vi "Timer.vi"(11 "Error_In":errorcluster, 13 "Timer_Select":T1=enum."Time_Out?") -> (4 "Time_Out?":bool, 15 "Error_Out":errorcluster)   [LabVIEW 2021]
doc: "Used for time out opertion."
uses:
  Controls/Timer_Select.ctl
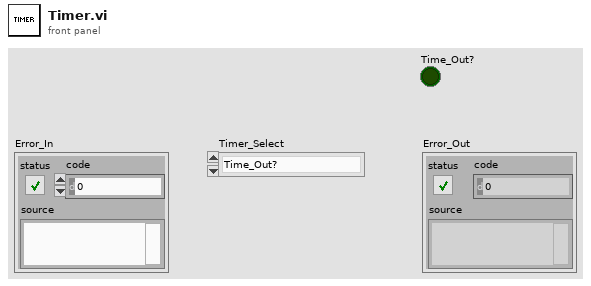
[diagram p1: front panel]
types:
  T1 = typedef "Timer_Select.ctl" = enum16{"Start_Timer", "Time_Out?", "Stop_Timer"}
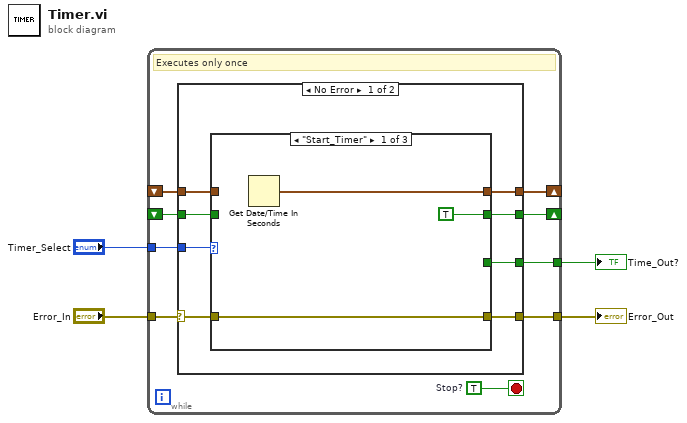
[diagram p0: block diagram]
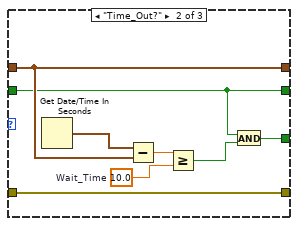
[diagram p2: hidden frame]
diagram:
  n1 = while {
    tunnel: "Timer_Select" -> [w13]
    shift-right: [w12] -> _
    shift-left: _ -> [w11]
    tunnel: [w10] -> w3
    tunnel: "Error_In" -> [w8]
    tunnel: [w7] -> w1
    shift-right: [w6] -> _
    shift-left: _ -> [w5]
    stop <- w9 stop-if-true
    w9 = TRUE  # Stop?
    # "Executes only once"
    n2 = case shown="No Error" w8 {
      selector: w8 -> [w17 w34]
      tunnel: w13 -> [w21 _]
      tunnel: [w20 w35] -> w12
      tunnel: w11 -> [w19 w35]
      tunnel: [w18 _] -> w10
      tunnel: [w16 w34] -> w7
      tunnel: [w15 _] -> w6
      tunnel: w5 -> [w14 _]
      frame No Error {
        n3 = case shown="\"Start_Timer\"" w21 {
          tunnel: [w23 w32 _] -> w20
          tunnel: w19 -> [_ w32 _]
          tunnel: [_ w26 _] -> w18
          tunnel: w17 -> [w24 w29 w33]
          tunnel: [w24 w29 w33] -> w16
          tunnel: [TRUE w25 _] -> w15
          tunnel: w14 -> [_ w25 _]
          frame "Start_Timer" {
            n4 = Get Date/Time In Seconds() -> (seconds since 1Jan1904=w23:timestamp)
          }
          frame "Time_Out?" {
            w27 = 10.0  # Wait_Time
            n5 = Get Date/Time In Seconds() -> (seconds since 1Jan1904=w28:timestamp)
            n6 = Subtract(x=w28, y=w32) -> (x-y=w31:dbl)
            n7 = Greater Or Equal?(x=w31, y=w27) -> (x >= y?=w30:bool)
            n8 = And(x=w25, y=w30) -> (x .and. y?=w26:bool)
          }
          frame "Stop_Timer" {
          }
        }
      }
      frame Error {
      }
    }
  }
  "Time_Out?" <- w3
  "Error_Out" <- w1
